vi "ADCP_Generate_Checksum_Raw_Packet.vi"(8 "error in (no error)":errorcluster, 10 "Raw Packet In":u8[](array[numeric]), 11 "ADCP in":refnum<class "ADCP.lvclass">) -> (0 "error out":errorcluster, 1 "Checksum":u8, 2 "Raw Packet Out":u8[](array[numeric]), 3 "ADCP out":refnum<class "ADCP.lvclass">)   [LabVIEW 2017, in "ADCP.lvclass"]
uses:
  ADCP.lvclass
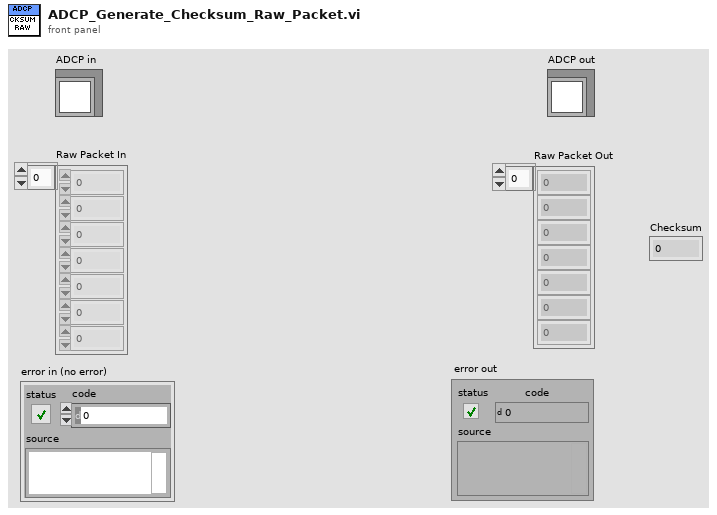
[diagram p1: front panel]
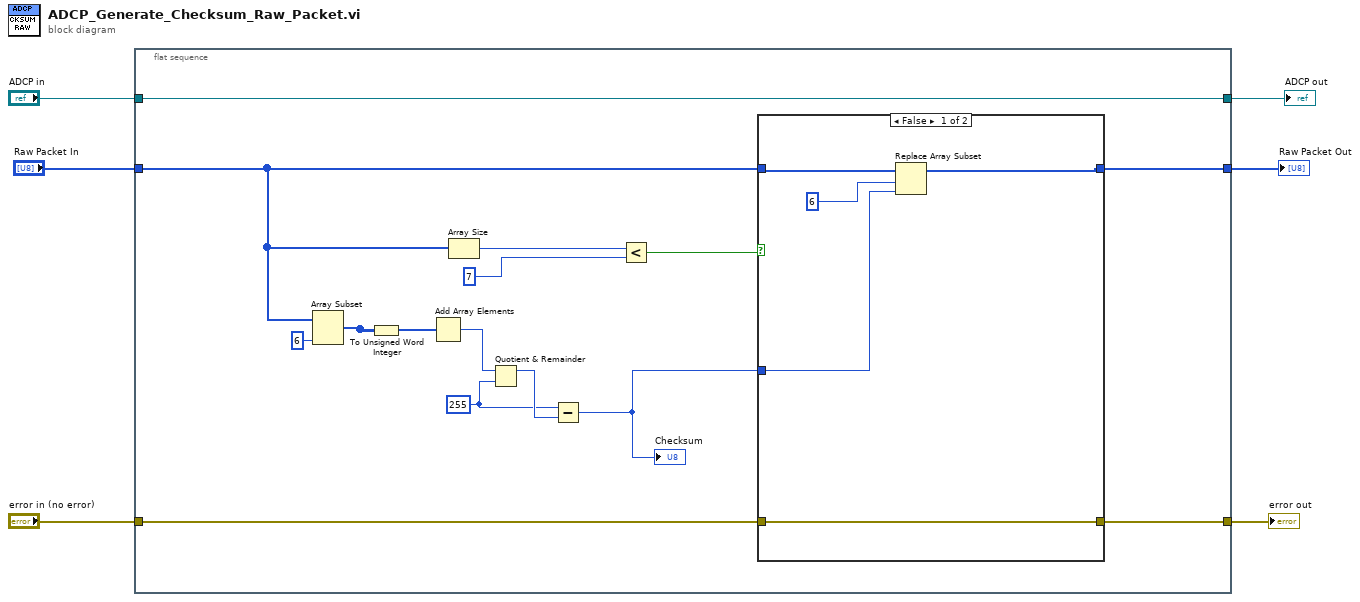
[diagram p0: block diagram]
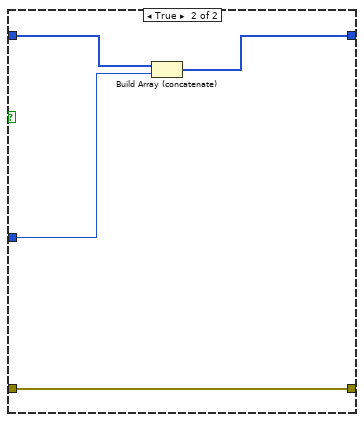
[diagram p2: hidden frame]
diagram:
  n1 = flat-sequence {
    tunnel: "error in (no error)" -> [w13]
    tunnel: [w12] -> w5
    tunnel: "ADCP in" -> [w20]
    tunnel: [w20] -> w3
    tunnel: "Raw Packet In" -> [w11]
    tunnel: [w10] -> w1
    frame #0 {
      w8 = u8 255 ("y")
      n2 = Array Subset(array=w11, length=6) -> (w18:u8[])  [unwired: 1 in]
      n3 = To Unsigned Word Integer(number=w18) -> ()  [unwired: 1 out]
      n4 = Add Array Elements(numeric array=w18) -> (sum=w17:u8)
      n5 = Array Size(array=w11) -> (size(s)=w16:i32)
      n6 = Quotient & Remainder(x=w17, y=w8) -> (x-y*floor(x/y)=w9:u8)  [unwired: 1 out]
      n7 = Subtract(x=w8, y=w9) -> (x-y=w7:u8)
      "Checksum" <- w7
      n8 = Less?(x=w16, y=7) -> (x < y?=w14:bool)
      n9 = case shown="False" w14 {
        tunnel: w13 -> [w25 w29]
        tunnel: [w25 w29] -> w12
        tunnel: w11 -> [w24 w28]
        tunnel: w7 -> [w22 w27]
        tunnel: [w21 w26] -> w10
        frame False {
          n10 = Replace Array Subset(array=w24, new element=w22, index=6) -> (w21:u8[])
        }
        frame True {
          n11 = Build Array (concatenate)(w28, w27) -> (w26:u8[])
        }
      }
    }
  }
  "ADCP out" <- w3
  "error out" <- w5
  "Raw Packet Out" <- w1
